vi "Create GUID.vi"(8 "error in (no error)":errorcluster) -> (0 "error out":errorcluster, 3 "Generated GUID":string)   [LabVIEW 2020, in "NIVS_Consolidated_CDW_MetaDataObj.lvclass"]
doc: "Create a new GUID (<B>G</B>lobally <B>U</B>nique <B>ID</B>entifier) string. A GUID enables VeriStand to identify an unique item."
uses:
  NIVS_Consolidated_CDW_MetaDataObj.lvclass
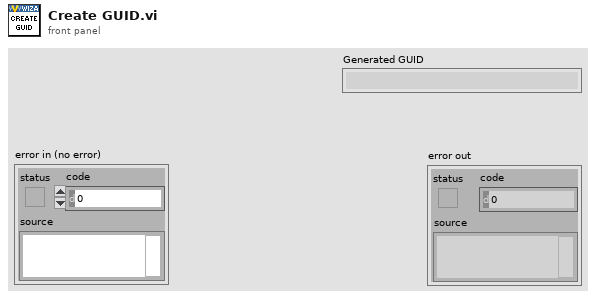
[diagram p1: front panel]
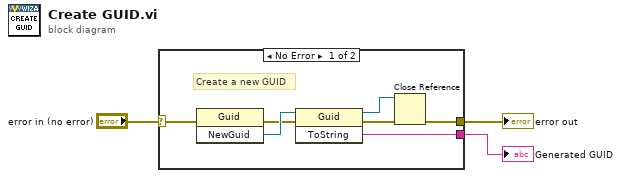
[diagram p0: block diagram]
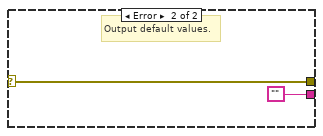
[diagram p2: hidden frame]
diagram:
  n1 = case shown="No Error" "error in (no error)" {
    selector: "error in (no error)" -> [w6 w12]
    tunnel: [w9 ""] -> w3
    tunnel: [w5 w12] -> w1
    frame No Error {
      # "Create a new GUID"
      n2 = invoke class="Guid" method="NewGuid"(error in=w6) -> (error out=w8:errorcluster, "NewGuid"=w10:refnum<k24>)  [unwired: 2 in, 1 out]
      n3 = invoke class="Guid" method="ToString"(reference=w10, error in=w8) -> (reference out=w4:refnum<k24>, error out=w7:errorcluster, "ToString"=w9:string)  [unwired: 1 in]
      n4 = Close Reference(reference=w4, error in (no error)=w7) -> (error out=w5:errorcluster)
    }
    frame Error {
      # "Output default values."
    }
  }
  "Generated GUID" <- w3
  "error out" <- w1
